vi "ini read-write.vi"(7 "action":T1, 8 "error in (no error)":errorcluster, 9 "ini entry descriptors":T2[](array[typedef]), 10 "values in":T4[](array[typedef]), 11 "configuration file path":path) -> (0 "error out":errorcluster, 2 "values out":T4[](array[typedef]), 3 "configuration file path out":path)   [LabVIEW 2014]
uses:
  type defs/ini entry value.ctl
  <vilib>/Utility/config.llb/NI_LVConfig.lvlib
  <vilib>/Utility/config.llb/Read Key (Boolean).vi
  <vilib>/Utility/config.llb/Write Key (Boolean).vi
  <vilib>/Utility/config.llb/Read Key (Double).vi
  <vilib>/Utility/config.llb/Write Key (Double).vi
  <vilib>/Utility/config.llb/Read Key (I32).vi
  <vilib>/Utility/config.llb/Write Key (I32).vi
  <vilib>/Utility/config.llb/Read Key (Path).vi
  <vilib>/Utility/config.llb/Write Key (Path).vi
  <vilib>/Utility/config.llb/Read Key (String).vi
  <vilib>/Utility/config.llb/Write Key (String).vi
  <vilib>/Utility/config.llb/Read Key (U32).vi
  <vilib>/Utility/config.llb/Write Key (U32).vi
  type defs/ini entry types.ctl
  type defs/ini entry.ctl
  type defs/ini file actions.ctl
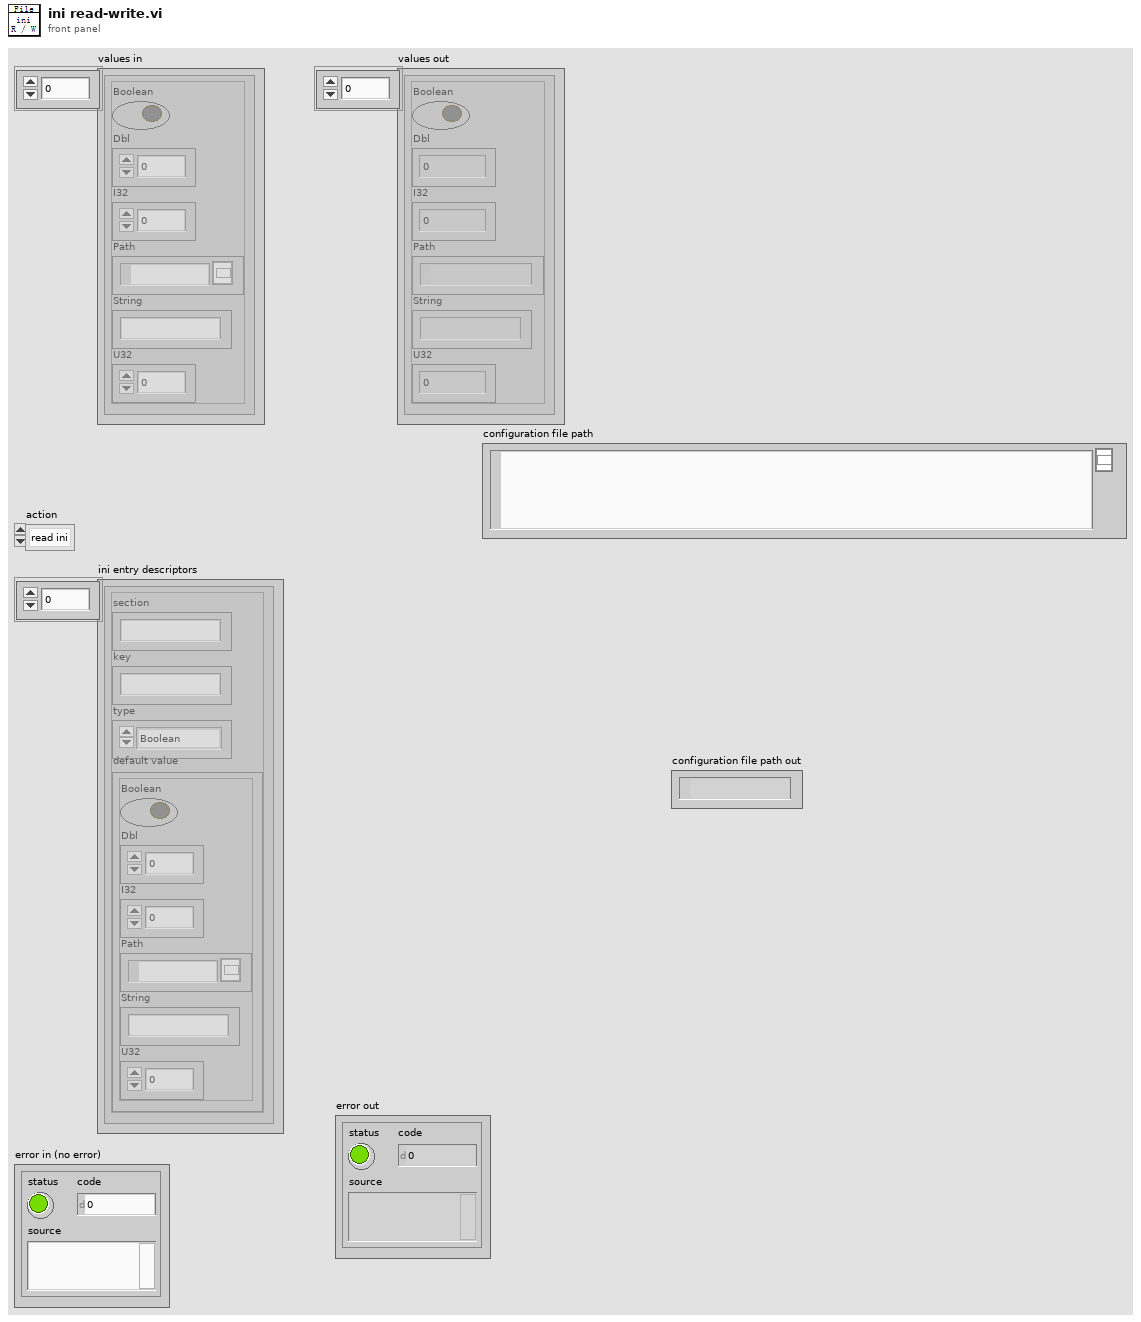
[diagram p1: front panel]
types:
  T1 = typedef "ini file actions.ctl" = enum16{"read ini", "write ini"}
  T2 = typedef "ini entry.ctl" = cluster{"section":string, "key":string, "type":T3, "default value":T4}
  T3 = typedef "ini entry types.ctl" = enum16{"Boolean", "Double", "I32", "Path", "String", "U32"}
  T4 = typedef "ini entry value.ctl" = cluster{"Boolean":bool, "Dbl":dbl, "I32":i32, "Path":path, "String":string, "U32":u32}
  T5 = typedef "NI_LVConfig.lvlib/Config Data RefNum.ctl" = refnum<k1>
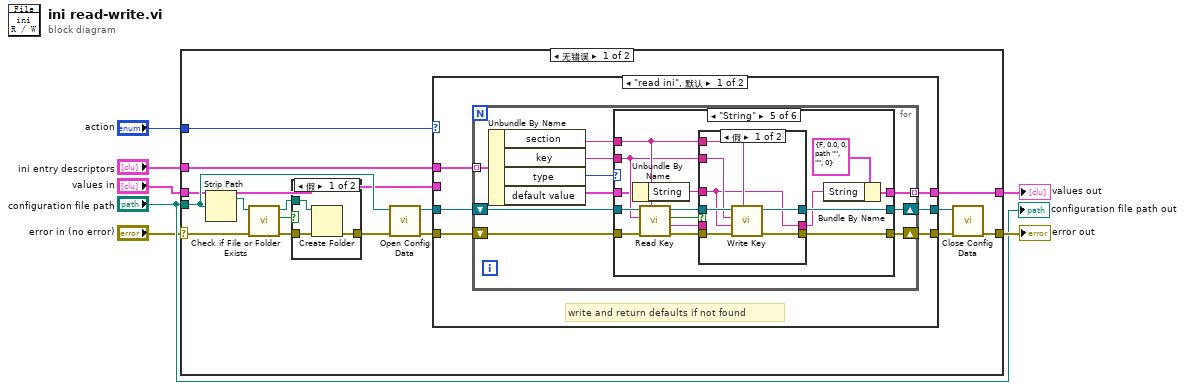
[diagram p0: block diagram]
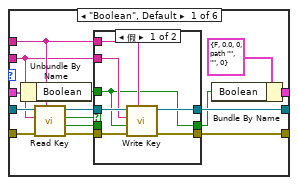
[diagram p3: hidden frame]
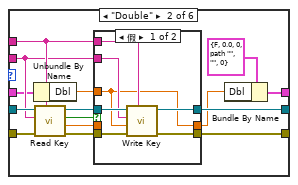
[diagram p5: hidden frame]
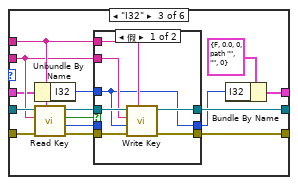
[diagram p7: hidden frame]
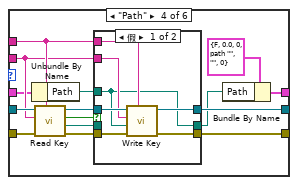
[diagram p9: hidden frame]
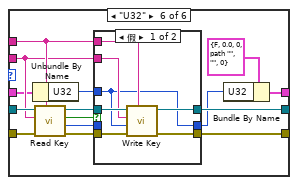
[diagram p12: hidden frame]
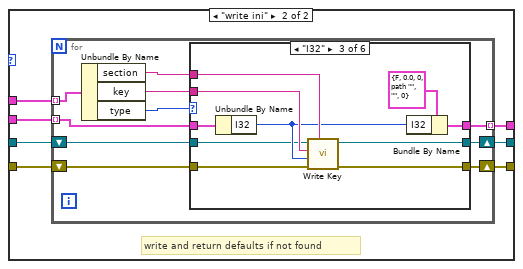
[diagram p14: hidden frame]
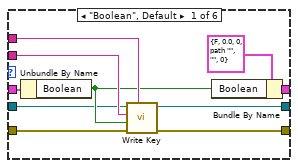
[diagram p15: hidden frame]
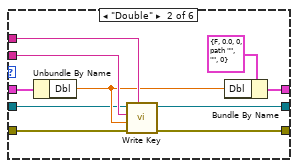
[diagram p16: hidden frame]
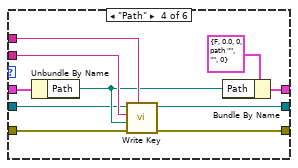
[diagram p17: hidden frame]
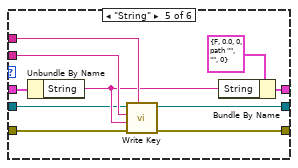
[diagram p18: hidden frame]
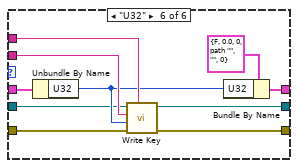
[diagram p19: hidden frame]
diagram:
  n1 = case shown="无错误" "error in (no error)" {
    selector: "error in (no error)" -> [w14 w272]
    tunnel: "action" -> [w23 _]
    tunnel: "ini entry descriptors" -> [w22 _]
    tunnel: "configuration file path" -> [w13 _]
    tunnel: [w8 w272] -> w5
    tunnel: [w10 w271] -> w6
    tunnel: "values in" -> [w9 w271]
    frame No Error {
      n2 = Strip Path(path=w13) -> (stripped path=w19:path)  [unwired: 1 out]
      n3 = call <vilib>:"Check if File or Folder Exists.vi"("error in (no error)"=w14, "path"=w19) -> ("error out"=w21:errorcluster, "file or folder exists?"=w17:bool, "dup path"=w18:path)  [unwired: 7 in]
      n4 = case shown="假" w17 {
        tunnel: w18 -> [w26 _]
        tunnel: [w25 w27] -> w20
        tunnel: w21 -> [w24 w27]
        frame False {
          n5 = Create Folder(path (use dialog)=w26, error in=w24) -> (error out=w25:errorcluster)  [unwired: 1 in, 2 out]
        }
        frame True {
        }
      }
      n6 = call <vilib>:"Open Config Data.vi"("error in (no error)"=w20, "configuration file path"=w13) -> ("error out"=w15:errorcluster, "refnum"=w16:T5)  [unwired: 7 in, 1 out]
      n7 = case shown="\"read ini\", 默认" w23 {
        tunnel: w22 -> [w33 w200]
        tunnel: [w32 w199] -> w12
        tunnel: w16 -> [w31 w198]
        tunnel: w15 -> [w30 w197]
        tunnel: [w29 w196] -> w11
        tunnel: [w28 w195] -> w10
        tunnel: w9 -> [_ w194]
        frame "read ini", Default {
          # "write and return defaults if not found"
          n8 = for {
            tunnel: w33 -> [w43] mode=indexing
            shift-right: [w37] -> w32
            shift-left: w31 -> [w38]
            shift-right: [w36] -> w29
            shift-left: w30 -> [w35]
            tunnel: [w34] -> w28 mode=indexing
            n9 = Unbundle By Name(w43) -> ("section"=w40:string, "key"=w39:string, "type"=w42:T3, "default value"=w41:T4)
            n10 = case shown="\"String\"" w42 {
              tunnel: w41 -> [w47 w72 w97 w122 w147 w172]
              tunnel: w40 -> [w49 w74 w99 w124 w149 w174]
              tunnel: w39 -> [w48 w73 w98 w123 w148 w173]
              tunnel: [w56 w81 w106 w131 w156 w181] -> w37
              tunnel: w38 -> [w55 w80 w105 w130 w155 w180]
              tunnel: [w54 w79 w104 w129 w154 w179] -> w36
              tunnel: w35 -> [w52 w77 w102 w127 w152 w177]
              tunnel: [w44 w69 w94 w119 w144 w169] -> w34
              frame "Boolean", Default {
                n11 = Unbundle By Name(w47) -> ("Boolean"=w46:bool)
                n12 = call-poly <vilib>:"Read Key.vi"("section"=w49, "error in (no error)"=w52, "key"=w48, "refnum"=w55) -> ("error out"=w53:errorcluster, "value"=w45:bool, "found?"=w58:bool, "refnum out"=w57:T5)  [unwired: 4 in]
                n13 = case shown="假" w58 {
                  tunnel: w57 -> [w64 w68]
                  tunnel: [w62 w68] -> w56
                  tunnel: [w61 w66] -> w54
                  tunnel: w53 -> [w60 w66]
                  tunnel: [w59 w67] -> w50
                  tunnel: w49 -> [w65 _]
                  tunnel: w48 -> [w63 _]
                  tunnel: w46 -> [w59 _]
                  tunnel: w45 -> [_ w67]
                  frame False {
                    n14 = call-poly <vilib>:"Write Key.vi"("section"=w65, "error in (no error)"=w60, "value"=w59, "key"=w63, "refnum"=w64) -> ("error out"=w61:errorcluster, "refnum out"=w62:T5)  [unwired: 4 in, 1 out]
                  }
                  frame True {
                  }
                }
                n15 = Bundle By Name(cluster=T4 {"Boolean"=FALSE, "Dbl"=0.0, "I32"=0, "Path"=path "", "String"="", "U32"=0}, "Boolean"=w50) -> (w44:T4)
              }
              frame "Double" {
                n16 = Unbundle By Name(w72) -> ("Dbl"=w71:dbl)
                n17 = call-poly <vilib>:"Read Key.vi"("section"=w74, "error in (no error)"=w77, "key"=w73, "refnum"=w80) -> ("error out"=w78:errorcluster, "value"=w70:dbl, "found?"=w83:bool, "refnum out"=w82:T5)  [unwired: 4 in]
                n18 = case shown="假" w83 {
                  tunnel: w82 -> [w89 w93]
                  tunnel: [w87 w93] -> w81
                  tunnel: [w86 w91] -> w79
                  tunnel: w78 -> [w85 w91]
                  tunnel: [w84 w92] -> w75
                  tunnel: w74 -> [w90 _]
                  tunnel: w73 -> [w88 _]
                  tunnel: w71 -> [w84 _]
                  tunnel: w70 -> [_ w92]
                  frame False {
                    n19 = call-poly <vilib>:"Write Key.vi"("section"=w90, "error in (no error)"=w85, "value"=w84, "key"=w88, "refnum"=w89) -> ("error out"=w86:errorcluster, "refnum out"=w87:T5)  [unwired: 4 in, 1 out]
                  }
                  frame True {
                  }
                }
                n20 = Bundle By Name(cluster=T4 {"Boolean"=FALSE, "Dbl"=0.0, "I32"=0, "Path"=path "", "String"="", "U32"=0}, "Dbl"=w75) -> (w69:T4)
              }
              frame "I32" {
                n21 = Unbundle By Name(w97) -> ("I32"=w96:i32)
                n22 = call-poly <vilib>:"Read Key.vi"("section"=w99, "error in (no error)"=w102, "key"=w98, "refnum"=w105) -> ("error out"=w103:errorcluster, "value"=w95:i32, "found?"=w108:bool, "refnum out"=w107:T5)  [unwired: 4 in]
                n23 = case shown="假" w108 {
                  tunnel: w107 -> [w114 w118]
                  tunnel: [w112 w118] -> w106
                  tunnel: [w111 w116] -> w104
                  tunnel: w103 -> [w110 w116]
                  tunnel: [w109 w117] -> w100
                  tunnel: w99 -> [w115 _]
                  tunnel: w98 -> [w113 _]
                  tunnel: w96 -> [w109 _]
                  tunnel: w95 -> [_ w117]
                  frame False {
                    n24 = call-poly <vilib>:"Write Key.vi"("section"=w115, "error in (no error)"=w110, "value"=w109, "key"=w113, "refnum"=w114) -> ("error out"=w111:errorcluster, "refnum out"=w112:T5)  [unwired: 4 in, 1 out]
                  }
                  frame True {
                  }
                }
                n25 = Bundle By Name(cluster=T4 {"Boolean"=FALSE, "Dbl"=0.0, "I32"=0, "Path"=path "", "String"="", "U32"=0}, "I32"=w100) -> (w94:T4)
              }
              frame "Path" {
                n26 = Unbundle By Name(w122) -> ("Path"=w121:path)
                n27 = call-poly <vilib>:"Read Key.vi"("section"=w124, "error in (no error)"=w127, "key"=w123, "refnum"=w130) -> ("error out"=w128:errorcluster, "value"=w120:path, "found?"=w133:bool, "refnum out"=w132:T5)  [unwired: 4 in]
                n28 = case shown="假" w133 {
                  tunnel: w132 -> [w139 w143]
                  tunnel: [w137 w143] -> w131
                  tunnel: [w136 w141] -> w129
                  tunnel: w128 -> [w135 w141]
                  tunnel: [w134 w142] -> w125
                  tunnel: w124 -> [w140 _]
                  tunnel: w123 -> [w138 _]
                  tunnel: w121 -> [w134 _]
                  tunnel: w120 -> [_ w142]
                  frame False {
                    n29 = call-poly <vilib>:"Write Key.vi"("section"=w140, "error in (no error)"=w135, "value"=w134, "key"=w138, "refnum"=w139) -> ("error out"=w136:errorcluster, "refnum out"=w137:T5)  [unwired: 4 in, 1 out]
                  }
                  frame True {
                  }
                }
                n30 = Bundle By Name(cluster=T4 {"Boolean"=FALSE, "Dbl"=0.0, "I32"=0, "Path"=path "", "String"="", "U32"=0}, "Path"=w125) -> (w119:T4)
              }
              frame "String" {
                n31 = Unbundle By Name(w147) -> ("String"=w146:string)
                n32 = call-poly <vilib>:"Read Key.vi"("section"=w149, "error in (no error)"=w152, "key"=w148, "refnum"=w155) -> ("error out"=w153:errorcluster, "value"=w145:string, "found?"=w158:bool, "refnum out"=w157:T5)  [unwired: 4 in]
                n33 = case shown="假" w158 {
                  tunnel: w157 -> [w164 w168]
                  tunnel: [w162 w168] -> w156
                  tunnel: [w161 w166] -> w154
                  tunnel: w153 -> [w160 w166]
                  tunnel: [w159 w167] -> w150
                  tunnel: w149 -> [w165 _]
                  tunnel: w148 -> [w163 _]
                  tunnel: w146 -> [w159 _]
                  tunnel: w145 -> [_ w167]
                  frame False {
                    n34 = call-poly <vilib>:"Write Key.vi"("section"=w165, "error in (no error)"=w160, "value"=w159, "key"=w163, "refnum"=w164) -> ("error out"=w161:errorcluster, "refnum out"=w162:T5)  [unwired: 4 in, 1 out]
                  }
                  frame True {
                  }
                }
                n35 = Bundle By Name(cluster=T4 {"Boolean"=FALSE, "Dbl"=0.0, "I32"=0, "Path"=path "", "String"="", "U32"=0}, "String"=w150) -> (w144:T4)
              }
              frame "U32" {
                n36 = Unbundle By Name(w172) -> ("U32"=w171:u32)
                n37 = call-poly <vilib>:"Read Key.vi"("section"=w174, "error in (no error)"=w177, "key"=w173, "refnum"=w180) -> ("error out"=w178:errorcluster, "value"=w170:u32, "found?"=w183:bool, "refnum out"=w182:T5)  [unwired: 4 in]
                n38 = case shown="假" w183 {
                  tunnel: w182 -> [w189 w193]
                  tunnel: [w187 w193] -> w181
                  tunnel: [w186 w191] -> w179
                  tunnel: w178 -> [w185 w191]
                  tunnel: [w184 w192] -> w175
                  tunnel: w174 -> [w190 _]
                  tunnel: w173 -> [w188 _]
                  tunnel: w171 -> [w184 _]
                  tunnel: w170 -> [_ w192]
                  frame False {
                    n39 = call-poly <vilib>:"Write Key.vi"("section"=w190, "error in (no error)"=w185, "value"=w184, "key"=w188, "refnum"=w189) -> ("error out"=w186:errorcluster, "refnum out"=w187:T5)  [unwired: 4 in, 1 out]
                  }
                  frame True {
                  }
                }
                n40 = Bundle By Name(cluster=T4 {"Boolean"=FALSE, "Dbl"=0.0, "I32"=0, "Path"=path "", "String"="", "U32"=0}, "U32"=w175) -> (w169:T4)
              }
            }
          }
        }
        frame "write ini" {
          # "write and return defaults if not found"
          n41 = for {
            tunnel: w200 -> [w210] mode=indexing
            shift-right: [w205] -> w199
            shift-left: w198 -> [w206]
            shift-right: [w204] -> w196
            shift-left: w197 -> [w203]
            tunnel: [w202] -> w195 mode=indexing
            tunnel: w194 -> [w201] mode=indexing
            n42 = Unbundle By Name(w210) -> ("section"=w208:string, "key"=w207:string, "type"=w209:T3)
            n43 = case shown="\"I32\"" w209 {
              tunnel: w201 -> [w215 w225 w235 w245 w255 w265]
              tunnel: w208 -> [w217 w227 w237 w247 w257 w267]
              tunnel: w207 -> [w216 w226 w236 w246 w256 w266]
              tunnel: [w220 w230 w240 w250 w260 w270] -> w205
              tunnel: w206 -> [w212 w221 w232 w241 w252 w262]
              tunnel: [w219 w229 w239 w249 w259 w269] -> w204
              tunnel: w203 -> [w211 w222 w231 w242 w251 w261]
              tunnel: [w213 w223 w233 w243 w253 w263] -> w202
              frame "Boolean", Default {
                n44 = Unbundle By Name(w215) -> ("Boolean"=w214:bool)
                n45 = call-poly <vilib>:"Write Key.vi"("section"=w217, "error in (no error)"=w211, "value"=w214, "key"=w216, "refnum"=w212) -> ("error out"=w219:errorcluster, "refnum out"=w220:T5)  [unwired: 4 in, 1 out]
                n46 = Bundle By Name(cluster=T4 {"Boolean"=FALSE, "Dbl"=0.0, "I32"=0, "Path"=path "", "String"="", "U32"=0}, "Boolean"=w214) -> (w213:T4)
              }
              frame "Double" {
                n47 = Unbundle By Name(w225) -> ("Dbl"=w224:dbl)
                n48 = call-poly <vilib>:"Write Key.vi"("section"=w227, "error in (no error)"=w222, "value"=w224, "key"=w226, "refnum"=w221) -> ("error out"=w229:errorcluster, "refnum out"=w230:T5)  [unwired: 4 in, 1 out]
                n49 = Bundle By Name(cluster=T4 {"Boolean"=FALSE, "Dbl"=0.0, "I32"=0, "Path"=path "", "String"="", "U32"=0}, "Dbl"=w224) -> (w223:T4)
              }
              frame "I32" {
                n50 = Unbundle By Name(w235) -> ("I32"=w234:i32)
                n51 = call-poly <vilib>:"Write Key.vi"("section"=w237, "error in (no error)"=w231, "value"=w234, "key"=w236, "refnum"=w232) -> ("error out"=w239:errorcluster, "refnum out"=w240:T5)  [unwired: 4 in, 1 out]
                n52 = Bundle By Name(cluster=T4 {"Boolean"=FALSE, "Dbl"=0.0, "I32"=0, "Path"=path "", "String"="", "U32"=0}, "I32"=w234) -> (w233:T4)
              }
              frame "Path" {
                n53 = Unbundle By Name(w245) -> ("Path"=w244:path)
                n54 = call-poly <vilib>:"Write Key.vi"("section"=w247, "error in (no error)"=w242, "value"=w244, "key"=w246, "refnum"=w241) -> ("error out"=w249:errorcluster, "refnum out"=w250:T5)  [unwired: 4 in, 1 out]
                n55 = Bundle By Name(cluster=T4 {"Boolean"=FALSE, "Dbl"=0.0, "I32"=0, "Path"=path "", "String"="", "U32"=0}, "Path"=w244) -> (w243:T4)
              }
              frame "String" {
                n56 = Unbundle By Name(w255) -> ("String"=w254:string)
                n57 = call-poly <vilib>:"Write Key.vi"("section"=w257, "error in (no error)"=w251, "value"=w254, "key"=w256, "refnum"=w252) -> ("error out"=w259:errorcluster, "refnum out"=w260:T5)  [unwired: 4 in, 1 out]
                n58 = Bundle By Name(cluster=T4 {"Boolean"=FALSE, "Dbl"=0.0, "I32"=0, "Path"=path "", "String"="", "U32"=0}, "String"=w254) -> (w253:T4)
              }
              frame "U32" {
                n59 = Unbundle By Name(w265) -> ("U32"=w264:u32)
                n60 = call-poly <vilib>:"Write Key.vi"("section"=w267, "error in (no error)"=w261, "value"=w264, "key"=w266, "refnum"=w262) -> ("error out"=w269:errorcluster, "refnum out"=w270:T5)  [unwired: 4 in, 1 out]
                n61 = Bundle By Name(cluster=T4 {"Boolean"=FALSE, "Dbl"=0.0, "I32"=0, "Path"=path "", "String"="", "U32"=0}, "U32"=w264) -> (w263:T4)
              }
            }
          }
        }
      }
      n62 = call <vilib>:"Close Config Data.vi"("error in (no error)"=w11, "refnum"=w12) -> ("error out"=w8:errorcluster)  [unwired: 8 in, 1 out]
    }
    frame Error {
    }
  }
  "values out" <- w6
  "error out" <- w5
  "configuration file path out" <- "configuration file path"
